vi "V C P condition set.vi"(0 "VISA resource name":refnum<visa-resource-name>, 1 "Voltege":dbl, 2 "Current":dbl, 3 "Power":dbl, 5 "error in (no error)":errorcluster, 6 "Channel  (1: CH1)":u16(ring)=1 items=["CH1"=1, "CH2"=2, "CH3"=3, "CH4"=4], 7 "V&C Logic Condition":enum16{"AND", "OR", "NONE"}(ring), 8 "Voltage Condition":enum16{">V", "<V", "=V", "NONE"}(ring), 9 "C&P Logic Condition":enum16{"AND", "OR", "NONE"}(ring), 10 "Current Condition":enum16{">C", "<C", "=C", "NONE"}(ring), 12 "Power Condition":enum16{">P", "<P", "=P", "NONE"}(ring)) -> (14 "VISA resource name out":refnum<visa-resource-name>, 19 "error out":errorcluster)   [LabVIEW 2020, in "GPP.lvlib"]
uses:
  GPP.lvlib
  Function/VISA_COMMON.ctl
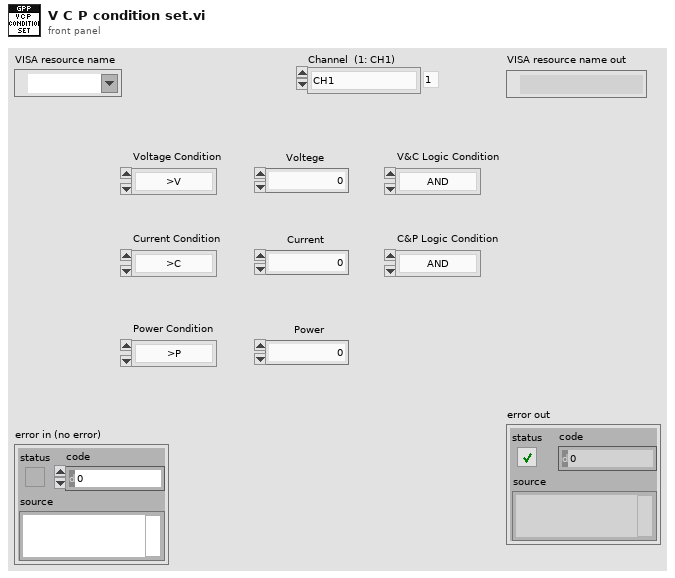
[diagram p1: front panel]
types:
  T1 = typedef "GPP.lvlib/VISA_COMMON.ctl" = enum16{"Initial", "Write CMD", "Read Result", "Read History", "Close"}
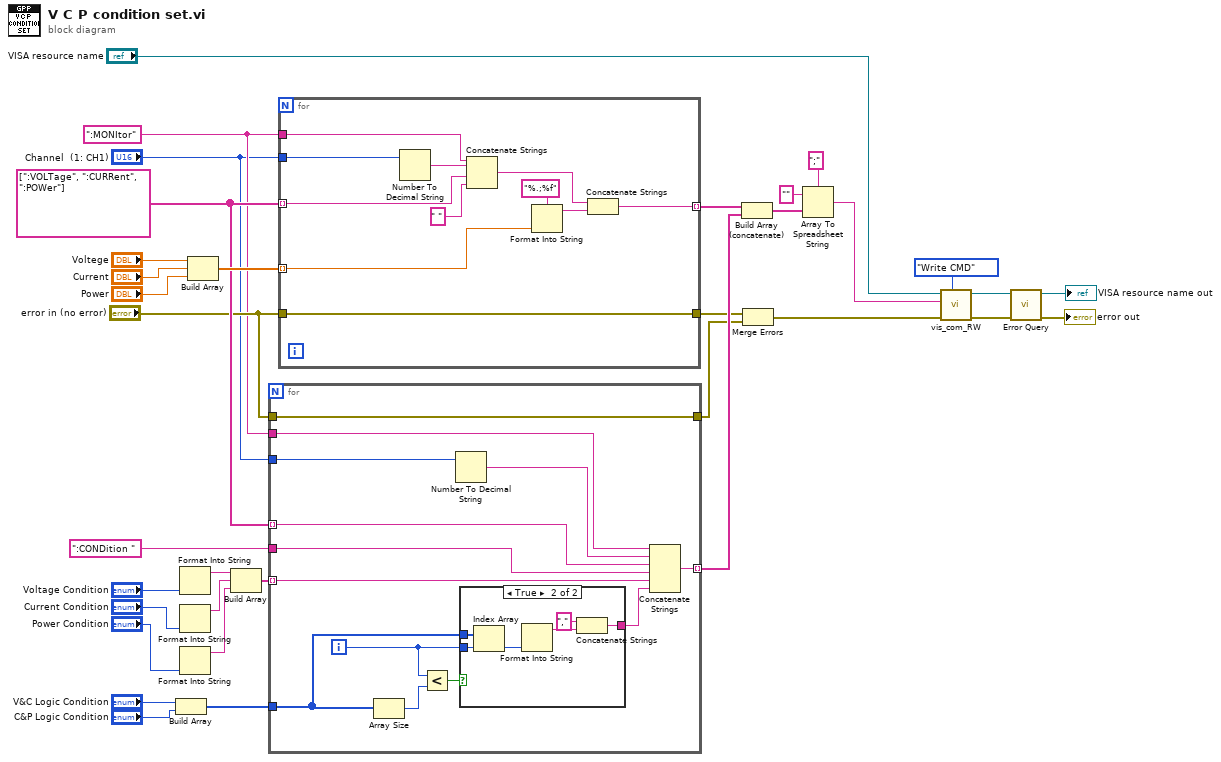
[diagram p0: block diagram]
diagram:
  w17 = ":MONItor"
  w22 = string[] [":VOLTage", ":CURRent", ":POWer"]
  n1 = Build Array("V&C Logic Condition", "C&P Logic Condition") -> (w23:enum16{"AND", "OR", "NONE"}[])
  n2 = Format Into String("Voltage Condition") -> (resulting string=w11:string)  [unwired: 3 in, 1 out]
  n3 = Format Into String("Current Condition") -> (resulting string=w10:string)  [unwired: 3 in, 1 out]
  n4 = Format Into String("Power Condition") -> (resulting string=w9:string)  [unwired: 3 in, 1 out]
  n5 = Build Array("Voltege", "Current", "Power") -> (w28:dbl[])
  n6 = Build Array(w11, w10, w9) -> (w8:string[])
  n7 = for {
    tunnel: [w41] -> w26 mode=indexing
    tunnel: w23 -> [w45]
    tunnel: w22 -> [w46] mode=indexing
    tunnel: "error in (no error)" -> [w40]
    tunnel: [w40] -> w19
    tunnel: w17 -> [w39]
    tunnel: "Channel  (1: CH1)" -> [w38]
    tunnel: ":CONDition " -> [w37]
    tunnel: w8 -> [w35] mode=indexing
    i -> [w36]
    n8 = Array Size(array=w45) -> (size(s)=w44:i32)
    n9 = Less?(x=w36, y=w44) -> (x < y?=w42:bool)
    n10 = Number To Decimal String(number=w38) -> (decimal integer string=w47:string)  [unwired: 1 in]
    n11 = case shown="True" w42 {
      tunnel: w45 -> [_ w50]
      tunnel: w36 -> [_ w49]
      tunnel: [_ w48] -> w43
      frame False {
      }
      frame True {
        n12 = Index Array(array=w50, index=w49) -> (element=w53:enum16{"AND", "OR", "NONE"})
        n13 = Format Into String(w53) -> (resulting string=w51:string)  [unwired: 3 in, 1 out]
        n14 = Concatenate Strings(",", w51) -> (w48:string)
      }
    }
    n15 = Concatenate Strings(w39, w47, w46, w37, w35, w43) -> (w41:string)
  }
  n16 = for {
    tunnel: [w60] -> w27 mode=indexing
    tunnel: w28 -> [w59] mode=indexing
    tunnel: w22 -> [w54] mode=indexing
    tunnel: "Channel  (1: CH1)" -> [w58]
    tunnel: "error in (no error)" -> [w57]
    tunnel: [w57] -> w20
    tunnel: w17 -> [w56]
    n17 = Number To Decimal String(number=w58) -> (decimal integer string=w63:string)  [unwired: 1 in]
    n18 = Concatenate Strings(w56, w63, w54, " " ("string")) -> (w64:string)
    n19 = Format Into String(format string="%.;%f", w59) -> (resulting string=w61:string)  [unwired: 2 in, 1 out]
    n20 = Concatenate Strings(w64, w61) -> (w60:string)
  }
  n21 = Build Array (concatenate)(w27, w26) -> (w2:string[])
  n22 = Merge Errors(w20, w19) -> (w18:errorcluster)
  n23 = Array To Spreadsheet String(delimiter (Tab)=";", array=w2, 3:"" ("format string")) -> (spreadsheet string=w1:string)
  n24 = call "vis_com_RW.vi"("Funciton"=VISA_COMMON."Write CMD", "error in (no error)"=w18, "CMD String"=w1, "VISA resource in"="VISA resource name") -> ("error out"=w4:errorcluster, "VISA resource out"=w5:refnum<visa-resource-name>)  [unwired: 5 in, 1 out]
  n25 = call "Error Query.vi"("error in (no error)"=w4, "VISA resource name"=w5) -> ("error out"=→"error out":errorcluster, "VISA resource name out"=→"VISA resource name out":refnum<visa-resource-name>)  [unwired: 6 in, 2 out]
